vi "Soft Serial-USB Host Keyboard.vi"   [LabVIEW 2014]
uses:
  QwaveSys_ESP8266/QwaveSys_ESP8266.lvlib
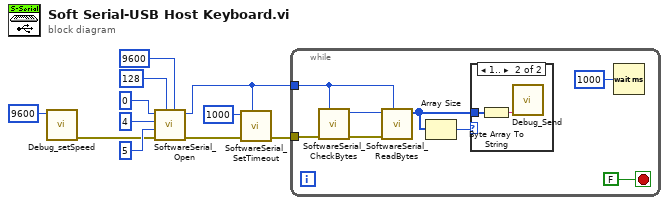
[diagram p0: block diagram]
diagram:
  n1 = call "Debug_setSpeed.vi"("Speed"=u32 9600) -> ("error out"=w6:errorcluster)  [unwired: 10 in]
  n2 = call "SoftwareSerial_Open.vi"("Speed"=u32 9600, "Buffer"=u8 128, "error in (no error)"=w6, "Tx"=u8 5, "Rx"=u8 4, "Interface (0-4)"=u8 0) -> ("error out"=w4:errorcluster, "Instance"=w2:u8)  [unwired: 4 in]
  n3 = call "SoftwareSerial_SetTimeout.vi"("Instance"=w2, "error in (no error)"=w4, "Timeout (ms)"=1000) -> ("error out"=w3:errorcluster)  [unwired: 8 in]
  n4 = while {
    tunnel: w3 -> [w17]
    tunnel: w2 -> [w14]
    stop <- FALSE stop-if-true
    n5 = call "SoftwareSerial_CheckBytes.vi"("Instance"=w14, "error in (no error)"=w17) -> ("error out"=w16:errorcluster, "Bytes"=w15:i32)  [unwired: 8 in]
    n6 = call "SoftwareSerial_ReadBytes.vi"("Instance"=w14, "error in (no error)"=w16, "Length"=w15) -> ("Data"=w13:u8[])  [unwired: 6 in, 2 out]
    n7 = Array Size(array=w13) -> (size(s)=w12:i32)
    n8 = case shown="1.." w12 {
      tunnel: w13 -> [_ w21]
      frame 0, Default {
      }
      frame 1.. {
        n9 = Byte Array To String(unsigned byte array=w21) -> (string=w20:string)
        n10 = call "Debug_Send.vi"("DATA"=w20) -> ()  [unwired: 11 in]
      }
    }
    n11 = Wait (ms)(milliseconds to wait=u32 1000) -> ()  [unwired: 1 out]
  }
